vi "Read From RoboteQ.vi"(8 "error in (no error)":errorcluster, 10 "channel number":u8, 11 "FPGA In":T1) -> (0 "error out":errorcluster, 1 "Read Bytes":string, 2 "Encoder Speed (RPM)":i32, 3 "FPGA Out":T1)   [LabVIEW 2012]
uses:
  901x DMA FPGA Reference.ctl
panel:
  out "Read Bytes 2":string
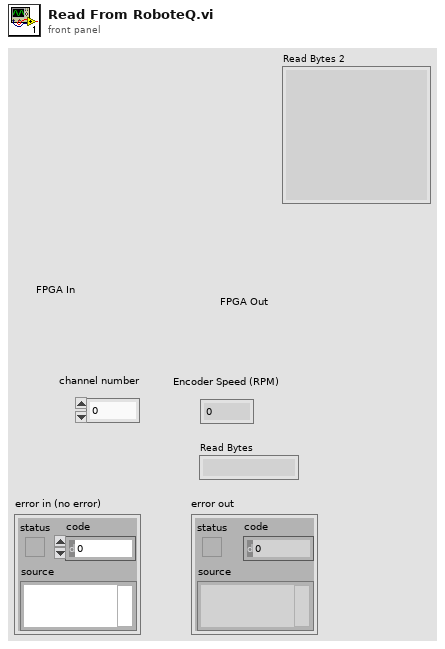
[diagram p1: front panel]
types:
  T1 = typedef "901x DMA FPGA Reference.ctl" = refnum<k20>
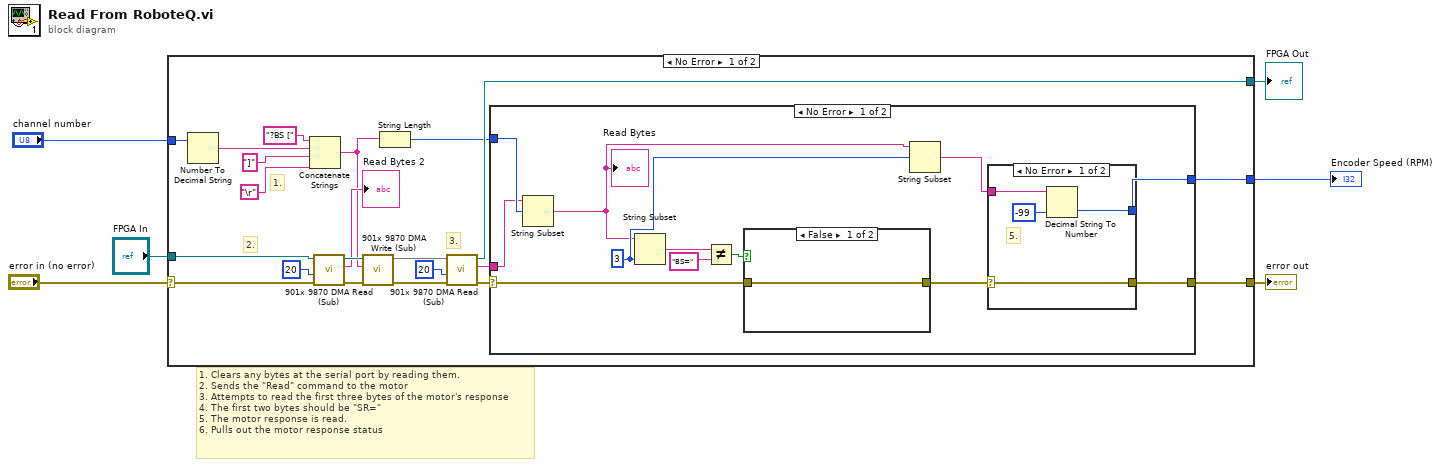
[diagram p0: block diagram]
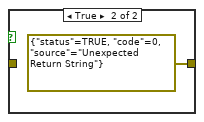
[diagram p2: hidden frame]
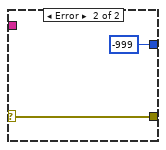
[diagram p3: hidden frame]
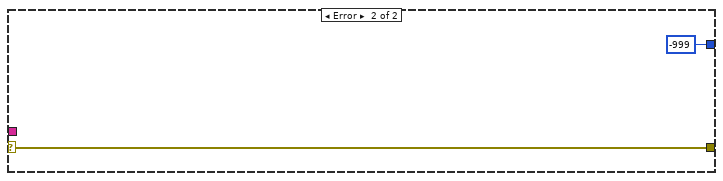
[diagram p4: hidden frame]
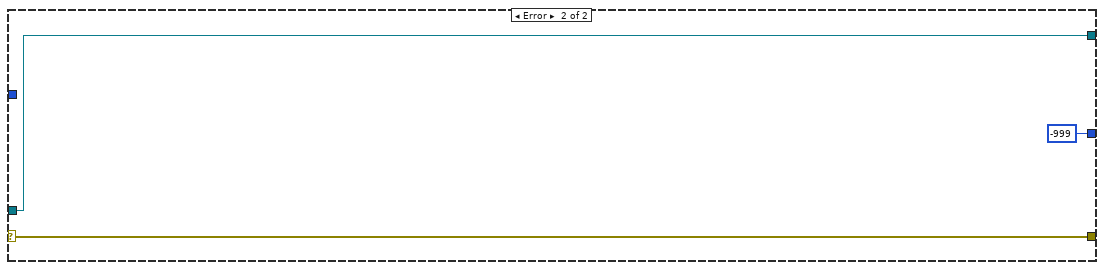
[diagram p5: hidden frame]
diagram:
  # "1. Clears any bytes at the serial port by reading them.\n2. Sends the \"Read\" command to the motor\n3. Attempts to read the first three bytes of the motor's response\n4. The first two bytes should be \"SR=\"\n5. The motor response is read.\n6. Pulls out the motor response status"
  n1 = case shown="No Error" "error in (no error)" {
    selector: "error in (no error)" -> [w11 w52]
    tunnel: [w26 w52] -> w5
    tunnel: [w27 -999 ("main battery\nvoltage (V)")] -> w4
    tunnel: "channel number" -> [w22 _]
    tunnel: "FPGA In" -> [w14 w50]
    tunnel: [w15 w50] -> w1
    frame No Error {
      # "3."
      # "2."
      # "1."
      n2 = Number To Decimal String(number=w22) -> (decimal integer string=w21:string)  [unwired: 1 in]
      n3 = Concatenate Strings("?BS [" ("string"), w21, "]" ("string"), "\r") -> (w8:string)
      n4 = call "901x 9870 DMA Read (Sub).vi"("error in"=w11, "Number of bytes"=20 ("Number of Bytes"), "FPGA In"=w14) -> ("error out"=w12:errorcluster, "Read Bytes"=→"Read Bytes 2":string, "FPGA Out"=w13:T1)  [unwired: 3 in, 3 out]
      n5 = call "901x 9870 DMA Write (Sub).vi"("error in"=w12, "Send Data"=w8, 11:w13) -> ("error out"=w17:errorcluster, 3:w18)  [unwired: 4 in, 3 out]
      n6 = String Length(string=w8) -> (length=w7:i32)
      n7 = call "901x 9870 DMA Read (Sub).vi"("error in"=w17, "Number of bytes"=u32 20 ("byte count"), "FPGA In"=w18) -> ("error out"=w20:errorcluster, "Read Bytes"=w19:string, "FPGA Out"=w15:T1)  [unwired: 3 in, 3 out]
      n8 = case shown="No Error" w20 {
        selector: w20 -> [w35 w49]
        tunnel: w19 -> [w32 _]
        tunnel: [w39 w49] -> w26
        tunnel: [w37 -999 ("main battery\nvoltage (V)")] -> w27
        tunnel: w7 -> [w33 _]
        frame No Error {
          w30 = 3 ("length (rest)")
          n9 = String Subset(string=w32, offset (0)=w33) -> (substring=w29:string)  [unwired: 1 in]
          "Read Bytes" <- w29
          n10 = String Subset(string=w29, length (rest)=w30) -> (substring=w31:string)  [unwired: 1 in]
          n11 = Not Equal?(x=w31, y="BS=" ("string")) -> (x != y?=w34:bool)
          n12 = case shown="False" w34 {
            tunnel: [w40 errorcluster {"status"=TRUE, "code"=0, "source"="Unexpected Return String"} ("error constant")] -> w36
            tunnel: w35 -> [w40 _]
            frame False {
            }
            frame True {
            }
          }
          n13 = String Subset(string=w29, offset (0)=w30) -> (substring=w28:string)  [unwired: 1 in]
          n14 = case shown="No Error" w36 {
            selector: w36 -> [w43 w47]
            tunnel: [w43 w47] -> w39
            tunnel: [w44 -999 ("main battery\nvoltage (V)")] -> w37
            tunnel: w28 -> [w42 _]
            frame No Error {
              # "5."
              n15 = Decimal String To Number(string=w42, default (0L)=-99 ("default (0 I32)")) -> (number=w44:i32)  [unwired: 1 in, 1 out]
            }
            frame Error {
            }
          }
        }
        frame Error {
        }
      }
    }
    frame Error {
    }
  }
  "error out" <- w5
  "Encoder Speed (RPM)" <- w4
  "FPGA Out" <- w1
